vi "获取公式存入关键参数.vi"(8 "error in (no error)":errorcluster caption="错误输入（无错误）", 9 "量程":u16, 10 "flowid":u16, 11 "id":u16) -> (0 "error out":errorcluster caption="错误输出", 3 "关键参数":T1)   [LabVIEW 2022 SP3, in "斯坦道CODcr.lvlib"]
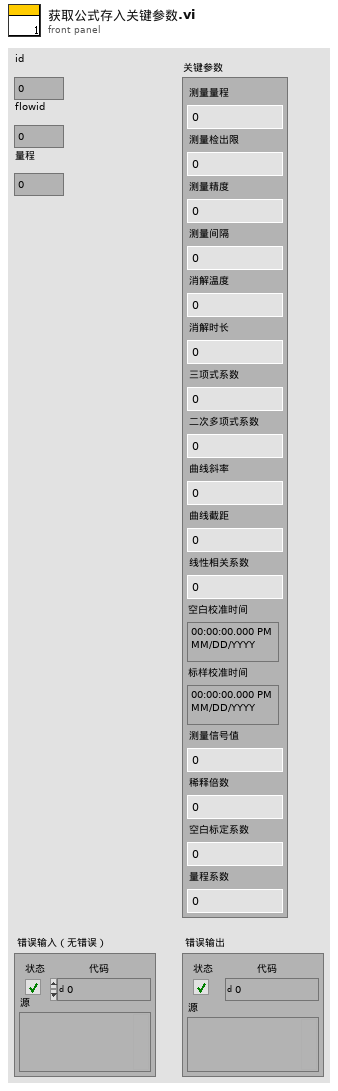
[diagram p1: front panel]
types:
  T1 = typedef "斯坦道CODcr.lvlib/关键参数.ctl" = cluster{"测量量程":sgl, "测量检出限":sgl, "测量精度":sgl, "测量间隔":sgl, "消解温度":sgl, "消解时长":sgl, "三项式系数":sgl, "二次多项式系数":sgl, "曲线斜率":sgl, "曲线截距":sgl, "线性相关系数":sgl, "空白校准时间":timestamp, "标样校准时间":timestamp, "测量信号值":sgl, "稀释倍数":sgl, "空白标定系数":sgl, "量程系数":sgl}
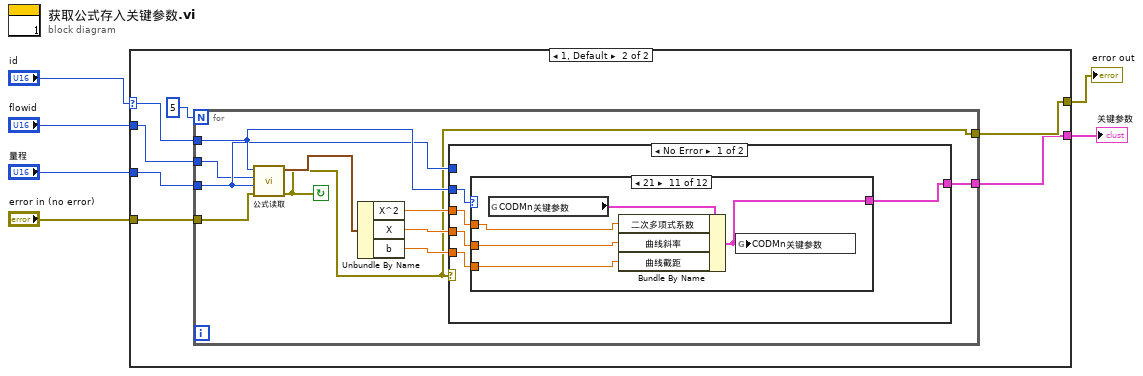
[diagram p0: block diagram]
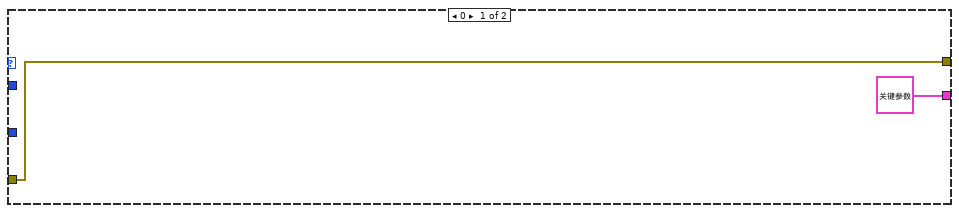
[diagram p2: hidden frame]
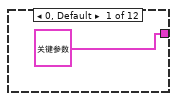
[diagram p3: hidden frame]
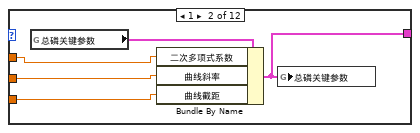
[diagram p4: hidden frame]
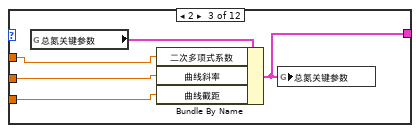
[diagram p5: hidden frame]
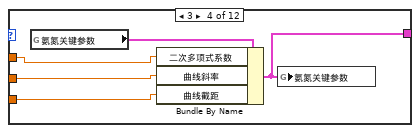
[diagram p6: hidden frame]
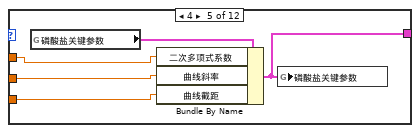
[diagram p7: hidden frame]
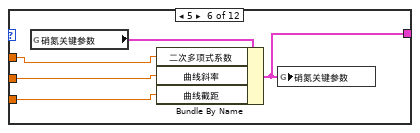
[diagram p8: hidden frame]
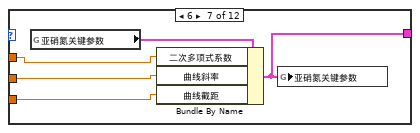
[diagram p9: hidden frame]
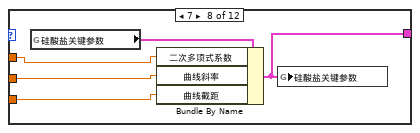
[diagram p10: hidden frame]
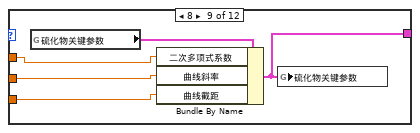
[diagram p11: hidden frame]
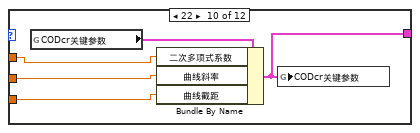
[diagram p12: hidden frame]
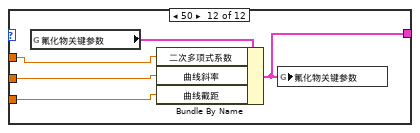
[diagram p13: hidden frame]
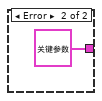
[diagram p14: hidden frame]
diagram:
  n1 = case shown="1, Default" "id" {
    selector: "id" -> [_ w10]
    tunnel: "flowid" -> [_ w14]
    tunnel: "量程" -> [_ w13]
    tunnel: "error in (no error)" -> [w8 w12]
    tunnel: [w8 w11] -> w3
    tunnel: [T1 {"测量量程"=0.0, "测量检出限"=0.0, "测量精度"=0.0, "测量间隔"=0.0, "消解温度"=0.0, "消解时长"=0.0, "三项式系数"=0.0, "二次多项式系数"=0.0, "曲线斜率"=0.0, "曲线截距"=0.0, "线性相关系数"=0.0, "空白校准时间"=timestamp(0 s since 1904-01-01), "标样校准时间"=timestamp(0 s since 1904-01-01), "测量信号值"=0.0, "稀释倍数"=0.0, "空白标定系数"=0.0, "量程系数"=0.0} ("氟化物关键参数") w9] -> w1
    frame 0 {
    }
    frame 1, Default {
      n2 = for {
        N: 5 -> [_]
        tunnel: w13 -> [w20]
        tunnel: w14 -> [w19]
        tunnel: w10 -> [w21]
        tunnel: w12 -> [w18]
        tunnel: [w17] -> w11
        tunnel: [w16] -> w9
        stop <- w17 continue-if-true
        n3 = call "公式读取.vi"("error in (no error)"=w18, "量程"=w20, "测量模式"=w19, "测量参数"=w21) -> ("error out"=w17:errorcluster, "公式"=w25:cluster{"X^2":dbl, "X":dbl, "b":dbl})  [unwired: 6 in]
        n4 = Unbundle By Name(w25) -> ("X^2"=w24:dbl, "X"=w23:dbl, "b"=w22:dbl)
        n5 = case shown="No Error" w17 {
          tunnel: w24 -> [w30 _]
          tunnel: w23 -> [w29 _]
          tunnel: w22 -> [w28 _]
          tunnel: w21 -> [w27 _]
          tunnel: w20 -> [_ _]
          tunnel: [w26 T1 {"测量量程"=0.0, "测量检出限"=0.0, "测量精度"=0.0, "测量间隔"=0.0, "消解温度"=0.0, "消解时长"=0.0, "三项式系数"=0.0, "二次多项式系数"=0.0, "曲线斜率"=0.0, "曲线截距"=0.0, "线性相关系数"=0.0, "空白校准时间"=timestamp(0 s since 1904-01-01), "标样校准时间"=timestamp(0 s since 1904-01-01), "测量信号值"=0.0, "稀释倍数"=0.0, "空白标定系数"=0.0, "量程系数"=0.0} ("氟化物关键参数")] -> w16
          frame No Error {
            n6 = case shown="21" w27 {
              tunnel: w30 -> [_ w35 w40 w45 w50 w55 w60 w65 w70 w75 w80 w85]
              tunnel: w29 -> [_ w34 w39 w44 w49 w54 w59 w64 w69 w74 w79 w84]
              tunnel: w28 -> [_ w33 w38 w43 w48 w53 w58 w63 w68 w73 w78 w83]
              tunnel: [T1 {"测量量程"=0.0, "测量检出限"=0.0, "测量精度"=0.0, "测量间隔"=0.0, "消解温度"=0.0, "消解时长"=0.0, "三项式系数"=0.0, "二次多项式系数"=0.0, "曲线斜率"=0.0, "曲线截距"=0.0, "线性相关系数"=0.0, "空白校准时间"=timestamp(0 s since 1904-01-01), "标样校准时间"=timestamp(0 s since 1904-01-01), "测量信号值"=0.0, "稀释倍数"=0.0, "空白标定系数"=0.0, "量程系数"=0.0} ("氟化物关键参数") w32 w37 w42 w47 w52 w57 w62 w67 w72 w77 w82] -> w26
              frame 0, Default {
              }
              frame 1 {
                n7 = global read "VAR总磷总氮全局变量.vi" "总磷关键参数"() -> (w36:T1)
                n8 = Bundle By Name(cluster=w36, "二次多项式系数"=w35, "曲线斜率"=w34, "曲线截距"=w33) -> (w32:T1)
                n9 = global write "VAR总磷总氮全局变量.vi" "总磷关键参数"(w32) -> ()
              }
              frame 2 {
                n10 = global read "VAR总磷总氮全局变量.vi" "总氮关键参数"() -> (w41:T1)
                n11 = Bundle By Name(cluster=w41, "二次多项式系数"=w40, "曲线斜率"=w39, "曲线截距"=w38) -> (w37:T1)
                n12 = global write "VAR总磷总氮全局变量.vi" "总氮关键参数"(w37) -> ()
              }
              frame 3 {
                n13 = global read "VAR总磷总氮全局变量.vi" "氨氮关键参数"() -> (w46:T1)
                n14 = Bundle By Name(cluster=w46, "二次多项式系数"=w45, "曲线斜率"=w44, "曲线截距"=w43) -> (w42:T1)
                n15 = global write "VAR总磷总氮全局变量.vi" "氨氮关键参数"(w42) -> ()
              }
              frame 4 {
                n16 = global read "VAR总磷总氮全局变量.vi" "磷酸盐关键参数"() -> (w51:T1)
                n17 = Bundle By Name(cluster=w51, "二次多项式系数"=w50, "曲线斜率"=w49, "曲线截距"=w48) -> (w47:T1)
                n18 = global write "VAR总磷总氮全局变量.vi" "磷酸盐关键参数"(w47) -> ()
              }
              frame 5 {
                n19 = global read "VAR总磷总氮全局变量.vi" "硝氮关键参数"() -> (w56:T1)
                n20 = Bundle By Name(cluster=w56, "二次多项式系数"=w55, "曲线斜率"=w54, "曲线截距"=w53) -> (w52:T1)
                n21 = global write "VAR总磷总氮全局变量.vi" "硝氮关键参数"(w52) -> ()
              }
              frame 6 {
                n22 = global read "VAR总磷总氮全局变量.vi" "亚硝氮关键参数"() -> (w61:T1)
                n23 = Bundle By Name(cluster=w61, "二次多项式系数"=w60, "曲线斜率"=w59, "曲线截距"=w58) -> (w57:T1)
                n24 = global write "VAR总磷总氮全局变量.vi" "亚硝氮关键参数"(w57) -> ()
              }
              frame 7 {
                n25 = global read "VAR总磷总氮全局变量.vi" "硅酸盐关键参数"() -> (w66:T1)
                n26 = Bundle By Name(cluster=w66, "二次多项式系数"=w65, "曲线斜率"=w64, "曲线截距"=w63) -> (w62:T1)
                n27 = global write "VAR总磷总氮全局变量.vi" "硅酸盐关键参数"(w62) -> ()
              }
              frame 8 {
                n28 = global read "VAR总磷总氮全局变量.vi" "硫化物关键参数"() -> (w71:T1)
                n29 = Bundle By Name(cluster=w71, "二次多项式系数"=w70, "曲线斜率"=w69, "曲线截距"=w68) -> (w67:T1)
                n30 = global write "VAR总磷总氮全局变量.vi" "硫化物关键参数"(w67) -> ()
              }
              frame 22 {
                n31 = global read "VAR总磷总氮全局变量.vi" "CODcr关键参数"() -> (w76:T1)
                n32 = Bundle By Name(cluster=w76, "二次多项式系数"=w75, "曲线斜率"=w74, "曲线截距"=w73) -> (w72:T1)
                n33 = global write "VAR总磷总氮全局变量.vi" "CODcr关键参数"(w72) -> ()
              }
              frame 21 {
                n34 = global read "VAR总磷总氮全局变量.vi" "CODMn关键参数"() -> (w81:T1)
                n35 = Bundle By Name(cluster=w81, "二次多项式系数"=w80, "曲线斜率"=w79, "曲线截距"=w78) -> (w77:T1)
                n36 = global write "VAR总磷总氮全局变量.vi" "CODMn关键参数"(w77) -> ()
              }
              frame 50 {
                n37 = global read "VAR总磷总氮全局变量.vi" "氟化物关键参数"() -> (w86:T1)
                n38 = Bundle By Name(cluster=w86, "二次多项式系数"=w85, "曲线斜率"=w84, "曲线截距"=w83) -> (w82:T1)
                n39 = global write "VAR总磷总氮全局变量.vi" "氟化物关键参数"(w82) -> ()
              }
            }
          }
          frame Error {
          }
        }
      }
    }
  }
  "error out" <- w3
  "关键参数" <- w1
